vi "FlatToRichrouteguide_RouteNote.vi"(5 "OutputClusterType":T1, 11 "InputCluster":T3) -> (3 "OutputCluster":T1)   [LabVIEW 2019, in "Generated_server.lvlib"]
uses:
  Generated_server.lvlib
  routeguide_RouteNote_Flat.ctl
  routeguide_Point_Flat.ctl
  routeguide_RouteNote.ctl
  routeguide_Point.ctl
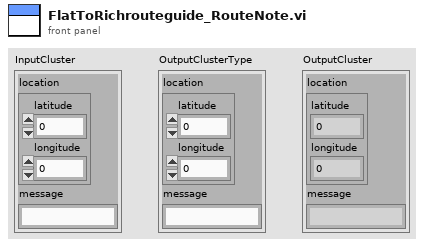
[diagram p1: front panel]
types:
  T1 = typedef "Generated_server.lvlib/routeguide_RouteNote.ctl" = cluster{"location":T2, "message":string}
  T2 = typedef "Generated_server.lvlib/routeguide_Point.ctl" = cluster{"latitude":i32, "longitude":i32}
  T3 = typedef "Generated_server.lvlib/routeguide_RouteNote_Flat.ctl" = cluster{"location":T4, "message":string}
  T4 = typedef "Generated_server.lvlib/routeguide_Point_Flat.ctl" = cluster{"latitude":i32, "longitude":i32}
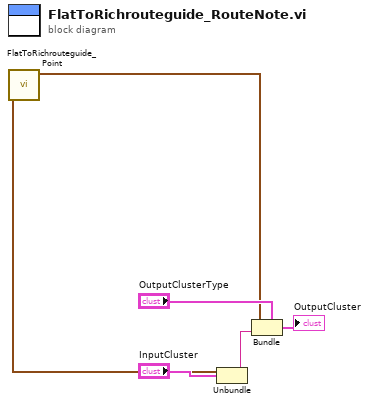
[diagram p0: block diagram]
diagram:
  n1 = Unbundle "Unbundle"("InputCluster") -> ("location"=w3:T4, "message"=w1:string)
  n2 = call "FlatToRichrouteguide_Point.vi"("InputCluster"=w3) -> ("OutputCluster"=w2:T2)  [unwired: 10 in]
  n3 = Bundle "Bundle"(cluster="OutputClusterType", "location"=w2, "message"=w1) -> (→"OutputCluster":T1)
